vi "Create.vi"(8 "error in (no error)":errorcluster, 9 "Getter VI Name":string, 10 "Setter VI Name":string, 11 "Class Type":refnum<class>) -> (0 "error out":errorcluster, 3 "Binding out":refnum<class "Binding.lvclass">)   [LabVIEW 2020, in "PropertyBinder.lvlib" / "Binding.lvclass"]
uses:
  Binding.lvclass
  PropertyBinder.lvlib
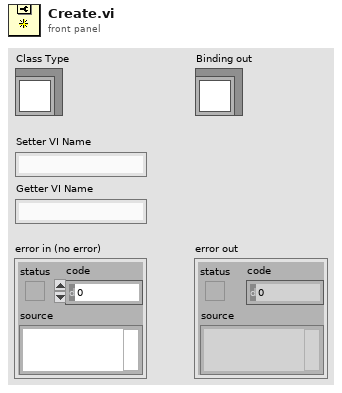
[diagram p1: front panel]
types:
  T1 = enum32{"invalid scope", "public", "private", "protected", "community"}
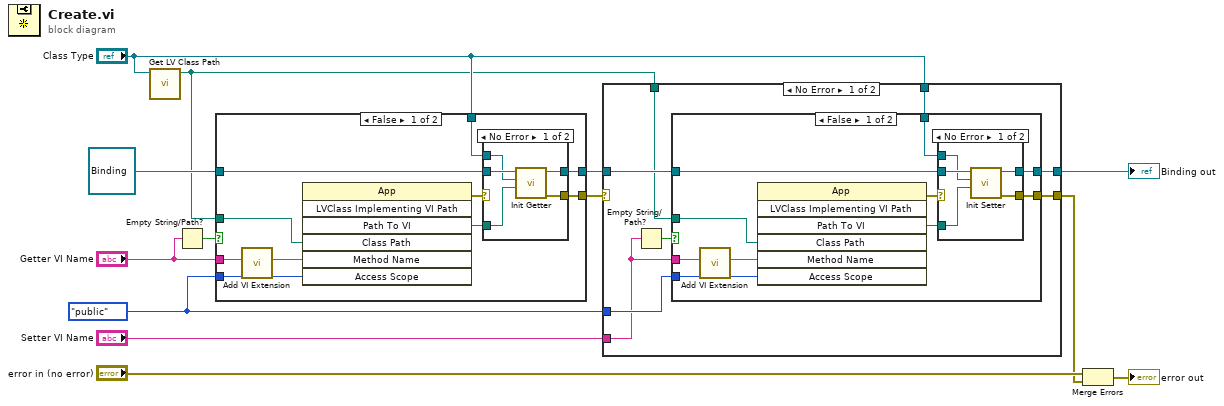
[diagram p0: block diagram]
diagram:
  w6 = T1."public" ("Access Scope")
  n1 = call <vilib>:"Get LV Class Path.vi"("object"="Class Type") -> ("class path"=w7:path)  [unwired: 9 in, 1 out]
  n2 = Empty String/Path?(string/path="Getter VI Name") -> (empty?=w11:bool)
  n3 = case shown="False" w11 {
    tunnel: w7 -> [w23 _]
    tunnel: "Getter VI Name" -> [w22 _]
    tunnel: w6 -> [w21 _]
    tunnel: refnum<class "Binding.lvclass"> refnum ("Binding in") -> [w18 w31]
    tunnel: "Class Type" -> [w17 _]
    tunnel: [w16 w31] -> w8
    tunnel: [w15 _] -> w3
    frame False {
      n4 = call "Add VI Extension.vi"("VI Name"=w22) -> ("VI Name with .vi"=w14:string)  [unwired: 10 in]
      n5 = invoke class="App" method="LVClass Implementing VI Path"("Class Path"=w23, "Method Name"=w14, "Access Scope"=w21) -> (error out=w20:errorcluster, "Path To VI"=w19:path)  [unwired: 4 in, 5 out]
      n6 = case shown="No Error" w20 {
        selector: w20 -> [_ w30]
        tunnel: w19 -> [w27 _]
        tunnel: w18 -> [w28 w29]
        tunnel: w17 -> [w26 _]
        tunnel: [w25 w29] -> w16
        tunnel: [w24 w30] -> w15
        frame No Error {
          n7 = call "Init Getter.vi"("Getter Path"=w27, "Class Type"=w26, "Binding in"=w28) -> ("error out"=w24:errorcluster, "Binding out"=w25:refnum<class "Binding.lvclass">)  [unwired: 7 in]
        }
        frame Error {
        }
      }
    }
    frame True {
    }
  }
  n8 = case shown="No Error" w3 {
    selector: w3 -> [_ w59]
    tunnel: "Class Type" -> [w39 _]
    tunnel: w8 -> [w38 w58]
    tunnel: w7 -> [w36 _]
    tunnel: w6 -> [w35 _]
    tunnel: "Setter VI Name" -> [w34 _]
    tunnel: [w33 w58] -> w4
    tunnel: [w32 w59] -> w1
    frame No Error {
      n9 = Empty String/Path?(string/path=w34) -> (empty?=w37:bool)
      n10 = case shown="False" w37 {
        tunnel: w36 -> [w49 _]
        tunnel: w34 -> [w48 _]
        tunnel: w35 -> [w47 _]
        tunnel: w38 -> [w44 w57]
        tunnel: [w43 w57] -> w33
        tunnel: [w42 _] -> w32
        tunnel: w39 -> [w41 _]
        frame False {
          n11 = call "Add VI Extension.vi"("VI Name"=w48) -> ("VI Name with .vi"=w40:string)  [unwired: 10 in]
          n12 = invoke class="App" method="LVClass Implementing VI Path"("Class Path"=w49, "Method Name"=w40, "Access Scope"=w47) -> (error out=w46:errorcluster, "Path To VI"=w45:path)  [unwired: 4 in, 5 out]
          n13 = case shown="No Error" w46 {
            selector: w46 -> [_ w56]
            tunnel: w45 -> [w53 _]
            tunnel: w44 -> [w54 w55]
            tunnel: w41 -> [w52 _]
            tunnel: [w51 w55] -> w43
            tunnel: [w50 w56] -> w42
            frame No Error {
              n14 = call "Init Setter.vi"("Setter Path"=w53, "Class Type"=w52, "Binding in"=w54) -> ("error out"=w50:errorcluster, "Binding out"=w51:refnum<class "Binding.lvclass">)  [unwired: 7 in]
            }
            frame Error {
            }
          }
        }
        frame True {
        }
      }
    }
    frame Error {
    }
  }
  "Binding out" <- w4
  n15 = Merge Errors("error in (no error)", w1) -> (→"error out":errorcluster)
